vi "poly_notify_name_by_name_multi.vi"(8 "error in":errorcluster caption="Error in (no error)", 9 "notifier names":string[](array[string]), 10 "name of caller in":string) -> (0 "error out":errorcluster, 4 "notified?":bool[](array[boolean]))   [LabVIEW 2015]
uses:
  ref_tools/polys/poly_control_ref_from_name_caller_multi.vi
  poly_notify_boolean_notifier_name.vi
  ref_tools/cores/core_ref_tools_eco.vi
  ref_tools/polys/poly_ref_tools_eco_plus.vi
  error_tools/cores/core_lvu_error_handler.vi
  ref_tools/polys/poly_control_ref_from_name_multi.vi
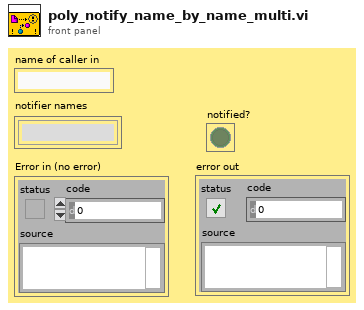
[diagram p1: front panel]
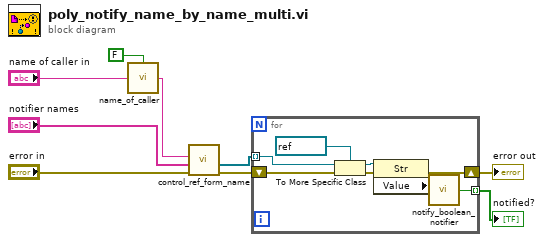
[diagram p0: block diagram]
diagram:
  n1 = call "name_of_caller.vi"("is in inlined vi? (F)"=FALSE, "name of caller in"="name of caller in") -> ("name of caller out"=w5:string)  [unwired: 2 in]
  n2 = call-poly "control_ref_form_name.vi"("error in"="error in", "control names"="notifier names", "name of caller in (your caller)"=w5) -> ("error out"=w7:errorcluster, "control refs"=w9:refnum<vi>[])  [unwired: 6 in, 1 out]
  n3 = for {
    tunnel: w9 -> [w17] mode=indexing
    tunnel: [w11] -> w1 mode=indexing
    shift-right: [w13] -> w6
    shift-left: w7 -> [w15]
    n4 = To More Specific Class(target class=refnum<vi> refnum ("String"), reference=w17, error in=w15) -> (specific class reference=w16:refnum<vi>, error out=w14:errorcluster)
    n5 = property class="Str"(reference=w16, error in=w14) -> (error out=w13:errorcluster, "Value"=w12:string)  [unwired: 1 out]
    n6 = call-poly "notify_boolean_notifier.vi"("notifier name"=w12) -> ("notified?"=w11:bool)  [unwired: 8 in]
  }
  "error out" <- w6
  "notified?" <- w1
